vi "WriteIQ_sglwfm.vi"(8 "error in (no error)":errorcluster, 10 "IQ wfm":waveform(csg), 11 "reference in":refnum<class "mmWave data.lvclass">) -> (0 "error out":errorcluster, 3 "reference out":refnum<class "mmWave data.lvclass">)   [LabVIEW 2019, in "mmWave data.lvclass"]
doc: "Writes IQ data to object"
uses:
  mmWave data.lvclass
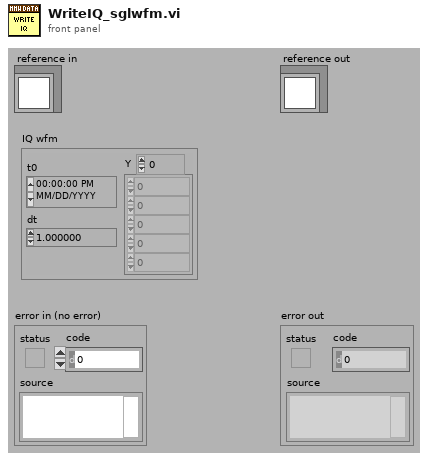
[diagram p1: front panel]
types:
  T1 = typedef "mmWave data.lvclass/ObjectAttributesRef.ctl" = refnum<data-value>
  T2 = typedef "mmWave data.lvclass/ObjectAttributes.ctl" = cluster{"MyAttribute":dbl, "size":i32}
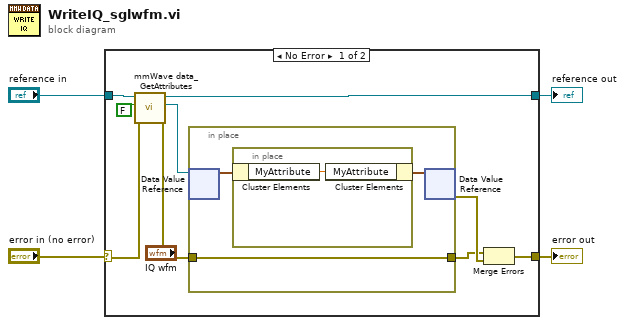
[diagram p0: block diagram]
diagram:
  n1 = case shown="No Error" "error in (no error)" {
    selector: "error in (no error)" -> [w8 w19]
    tunnel: [w13 w19] -> w3
    tunnel: [w6 w18] -> w1
    tunnel: "reference in" -> [w10 w18]
    frame No Error {
      n2 = call "mmWave data_GetAttributes.vi"("error in (no error)"=w8, "return data? (T)"=FALSE, "reference in"=w10) -> ("error out"=w7:errorcluster, "attributes ref"=w5:T1, "reference out"=w6:refnum<class "mmWave data.lvclass">)  [unwired: 5 in, 1 out]
      n3 = in-place {
        in-place-border: w7 -> [w14]
        in-place-border: [w14] -> w11
        n4 = in-place-dvr #1(w5) -> (w15:T2)  [unwired: 1 out]
        n5 = in-place {
          n6 = in-place-cluster #2(w15) -> ("MyAttribute"=w17:dbl)
          n7 = in-place-cluster #2("MyAttribute"=w17) -> (w16:T2)
        }
        n8 = in-place-dvr #1(w16) -> (w12:errorcluster)  [unwired: 1 out]
      }
      n9 = Merge Errors(w11, w12) -> (w13:errorcluster)
    }
    frame Error {
    }
  }
  "error out" <- w3
  "reference out" <- w1
